vi "get device channel.vi"(7 "device type (LAN)":T1=enum."LAN", 8 "error in (no error)":errorcluster, 11 "channel index (1)":u8=1) -> (0 "error out":errorcluster, 3 "channel":u16 format="%x")   [LabVIEW 2024, in "atsj peakcan basic.lvlib"]
doc: "Gets a PeakCAN channel for a given device type's <b>channel index</b>."
uses:
  atsj peakcan basic.lvlib
  device type.ctl
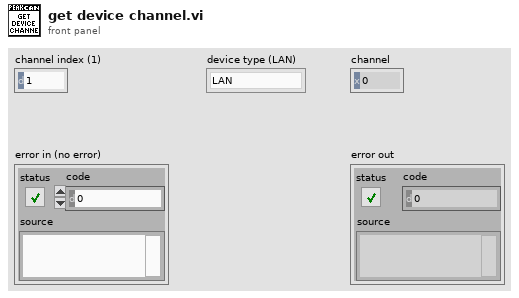
[diagram p1: front panel]
types:
  T1 = typedef "atsj peakcan basic.lvlib/device type.ctl" = enum8{"ISA", "DNG", "PCI", "USB", "PCC", "LAN"}
  T2 = typedef "atsj peakcan basic.lvlib/channel info.ctl" = cluster{"upper channel limit":u8, "lower channel limit":u8, "channel base":u16}
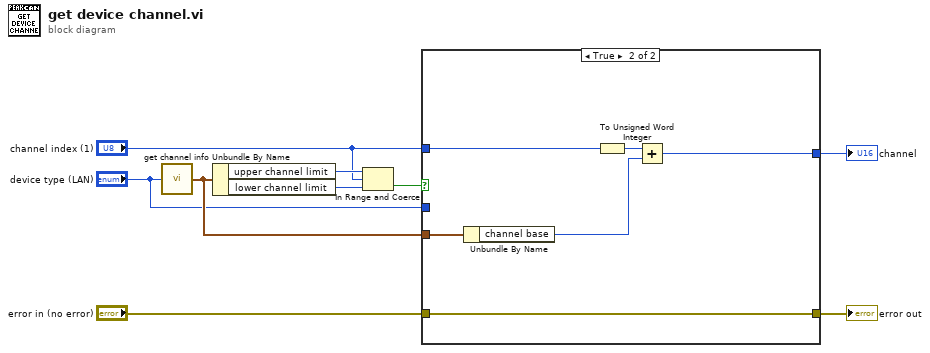
[diagram p0: block diagram]
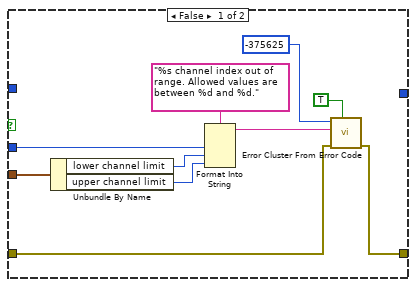
[diagram p2: hidden frame]
diagram:
  n1 = call "get channel info.vi"("device type"="device type (LAN)") -> ("device channel spec"=w2:T2)
  n2 = Unbundle By Name(w2) -> ("upper channel limit"=w5:u8, "lower channel limit"=w4:u8)
  n3 = In Range and Coerce(upper limit=w5, x="channel index (1)", lower limit=w4) -> (In Range?=w6:bool)  [unwired: 1 out]
  n4 = case shown="True" w6 {
    tunnel: "error in (no error)" -> [w17 w25]
    tunnel: [w16 w25] -> w8
    tunnel: "channel index (1)" -> [_ w24]
    tunnel: [_ w22] -> w7
    tunnel: w2 -> [w12 w21]
    tunnel: "device type (LAN)" -> [w13 _]
    frame False {
      n5 = Unbundle By Name(w12) -> ("lower channel limit"=w11:u8, "upper channel limit"=w10:u8)
      n6 = Format Into String(format string="%s channel index out of range. Allowed values are between %d and %d.", w13, w11, w10) -> (resulting string=w14:string)  [unwired: 2 in, 1 out]
      n7 = call <vilib>:"Error Cluster From Error Code.vi"("show call chain? (False)"=TRUE, "error in (no error)"=w17, "error message (\"\")"=w14, "error code (0)"=-375625) -> ("error out"=w16:errorcluster)  [unwired: 5 in]
    }
    frame True {
      n8 = Unbundle By Name(w21) -> ("channel base"=w20:u16)
      n9 = To Unsigned Word Integer(number=w24) -> (unsigned 16bit integer=w23:u16)
      n10 = Add(x=w23, y=w20) -> (x+y=w22:u16)
    }
  }
  "error out" <- w8
  "channel" <- w7
